vi "Select App.vi"(8 "error in (no error)":errorcluster, 11 "GWebAppArrayPanel in":refnum<class "GWebAppArrayPanel.lvclass">) -> (0 "error out":errorcluster, 3 "GWebAppArrayPanel out":refnum<class "GWebAppArrayPanel.lvclass">)   [LabVIEW 2020, in "PicoG-App.lvlib" / "GWebAppArrayPanel.lvclass"]
uses:
  GWebAppArrayPanel.lvclass
  GWebAppArrayPanel.lvclass/GWebAppArrayPanel.ctl
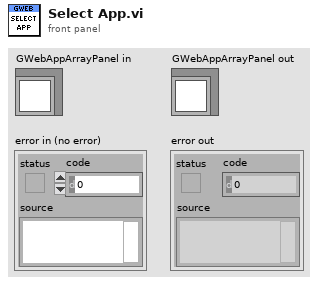
[diagram p1: front panel]
types:
  T1 = typedef "PicoG-App.lvlib/GWebAppArrayPanel.lvclass/Ref Data.ctl" = cluster{"App":refnum<class "ViaApp.lvclass">}
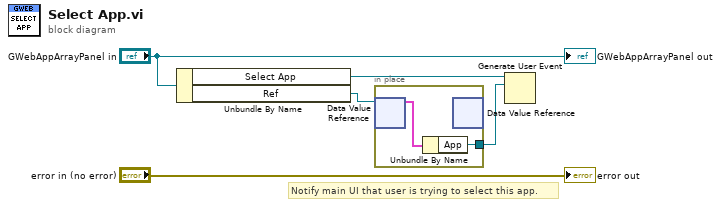
[diagram p0: block diagram]
diagram:
  # "Notify main UI that user is trying to select this app."
  n1 = Unbundle By Name("GWebAppArrayPanel in") -> ("Select App"=w2:refnum<user-event>, "Ref"=w4:refnum<data-value>)
  n2 = in-place {
    in-place-border: [w6] -> w3
    n3 = in-place-dvr #1(w4) -> (w7:T1)  [unwired: 1 out]
    n4 = Unbundle By Name(w7) -> ("App"=w6:refnum<class "ViaApp.lvclass">)
    n5 = in-place-dvr #1() -> ()  [unwired: 1 in, 2 out]
  }
  n6 = Generate User Event(user event=w2, event data cluster=w3) -> ()  [unwired: 2 in, 2 out]
  "error out" <- "error in (no error)"
  "GWebAppArrayPanel out" <- "GWebAppArrayPanel in"
